vi "rgb to grayscale single-threaded.vi"(7 "Depth?":bool, 8 "error in (no error)":errorcluster, 10 "Processing Params":T1, 11 "Image In":T2) -> (0 "error out":errorcluster, 2 "Depth Values":dbl[][](array[numeric]), 3 "Image Out":T2)   [LabVIEW 2018]
uses:
  <vilib>/vision/Image Controls.llb/IMAQ Image.ctl
  Processing Params STYP.ctl
  Pixel Data STYP.ctl
  Coordinate STYP.ctl
  Floating Pixel Data STYP.ctl
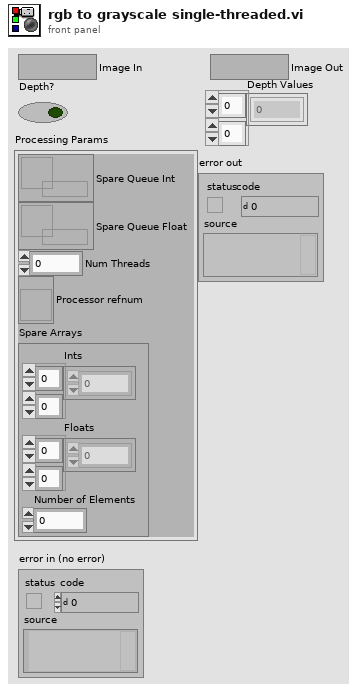
[diagram p1: front panel]
types:
  T1 = typedef "Processing Params STYP.ctl" = cluster{"Spare Queue Int":refnum<queue>, "Spare Queue Float":refnum<queue>, "Num Threads":i32, "Processor refnum":refnum<vi>, "Spare Arrays":cluster{"Ints":u8[][], "Floats":dbl[][], "Number of Elements":i32}}
  T2 = typedef "IMAQ Image.ctl" = refnum<image>
  T3 = typedef "Image Type" = u32
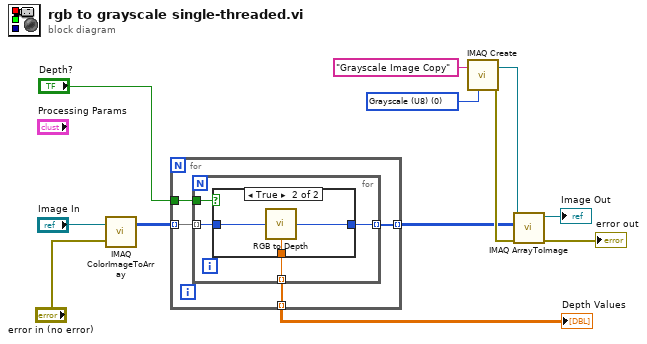
[diagram p0: block diagram]
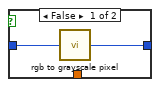
[diagram p2: hidden frame]
diagram:
  w3 = T3 0 items=["Grayscale (U8)", "Grayscale (I16)", "Grayscale (SGL)", "Complex (CSG)", "RGB (U32)", "HSL (U32)", "RGB (U64)", "Grayscale (U16)"] ("t")
  n1 = call "IMAQ ColorImageToArray"("Image"="Image In", "error in (no error)"="error in (no error)") -> ("Image Pixels (U32)"=w5:u32[][])  [unwired: 2 in, 2 out]
  n2 = for {
    tunnel: w5 -> [w16] mode=indexing
    tunnel: [w15] -> w2 mode=indexing
    tunnel: "Depth?" -> [w14]
    tunnel: [w13] -> w1 mode=indexing
    n3 = for {
      tunnel: w16 -> [w20] mode=indexing
      tunnel: [w19] -> w15 mode=indexing
      tunnel: w14 -> [w18]
      tunnel: [w17] -> w13 mode=indexing
      n4 = case shown="True" w18 {
        tunnel: w20 -> [w22 w25]
        tunnel: [w21 w24] -> w19
        tunnel: [_ w23] -> w17
        frame False {
          n5 = call "rgb to grayscale pixel.vi"("Color (U32)"=w22) -> ("Grayscale (U8)"=w21:u8)  [unwired: 14 in]
        }
        frame True {
          n6 = call "RGB to Depth.vi"("RGB"=w25) -> ("Depth Pixel"=w24:u8, "Depth"=w23:dbl)  [unwired: 13 in]
        }
      }
    }
  }
  "Depth Values" <- w1
  n7 = call "IMAQ Create"("Image Name"="Grayscale Image Copy", "Image Type"=w3) -> ("New Image"=w9:T2, "error out"=w8:errorcluster)  [unwired: 3 in]
  n8 = call "IMAQ ArrayToImage"("error in (no error)"=w8, "Image Pixels (U8)"=w2, "Image"=w9) -> ("error out"=→"error out":errorcluster, "Image Out"=→"Image Out":T2)  [unwired: 7 in]
